vi "Simple Button Lamp Example.vi"() -> ()   [LabVIEW 2018]
uses:
  Lamp/Lamp.lvclass
  Button/Button.lvclass
  Button/Button.lvclass/Button.ctl
  Button/Set Button Pressed.vi
  SwitchableDevice_interface/SwitchableDevice.lvclass
panel:
  out "Lamp":bool
  in  "Button":bool
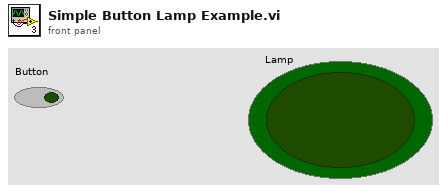
[diagram p1: front panel]
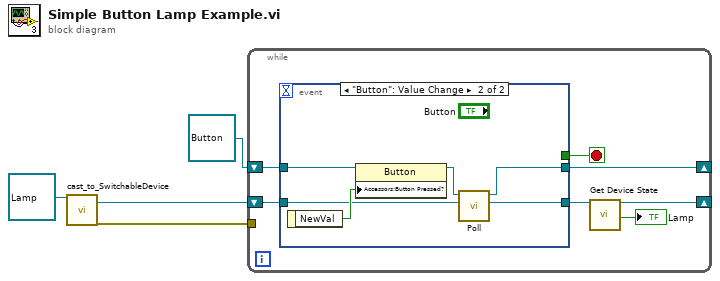
[diagram p0: block diagram]
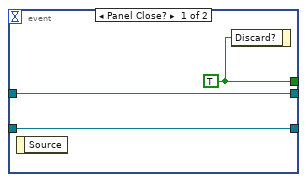
[diagram p2: hidden frame]
diagram:
  n1 = call "cast_to_SwitchableDevice.vi"("Object in"=refnum<class "Lamp.lvclass"> refnum ("Lamp.lvclass")) -> ("Interface_object out"=w2:refnum<class "SwitchableDevice.lvclass">, "error out"=w1:errorcluster)  [unwired: 17 in]
  n2 = while {
    shift-right: [w8] -> _
    shift-left: refnum<class "Button.lvclass"> refnum ("Button in") -> [w10]
    shift-right: [w6] -> _
    shift-left: w2 -> [w9]
    tunnel: w1 -> [_]
    stop <- w11 stop-if-true
    n3 = event shown="[1] \"Button\": Value Change" {
      selector: _ -> [_ _]
      dyn-events: _ -> [_ _]
      timeout: _ -> [_ _]
      tunnel: [w14 _] -> w11
      tunnel: w10 -> [w13 w20]
      tunnel: w9 -> [w12 w17]
      tunnel: [w13 w16] -> w8
      tunnel: [w12 w15] -> w7
      event Panel Close? {
        w14 = TRUE ("Discard?")
        n4 = event-data() -> ()  [unwired: 1 in, 1 out]
        n5 = event-data("Discard?"=w14) -> ()  [unwired: 1 in, 1 out]
      }
      event "Button": Value Change {
        n6 = event-data() -> ("NewVal"=w18:bool)  [unwired: 1 in]
        n7 = property class="Button"(reference=w20, "Accessors:Button Pressed?"=w18) -> (reference out=w19:refnum<class "Button.lvclass">)  [unwired: 1 in, 1 out]
        n8 = call-dynamic "Poll.vi"("Switchable Device in"=w17, "Button in"=w19) -> ("Switchable Device out"=w15:refnum<class "SwitchableDevice.lvclass">, "Button out"=w16:refnum<class "Button.lvclass">)  [unwired: 7 in, 1 out]
      }
    }
    n9 = call "Get Device State.vi"("Interface_object in"=w7) -> ("Interface_object out"=w6:refnum<class "SwitchableDevice.lvclass">, "Device State"=→"Lamp":bool)  [unwired: 16 in, 1 out]
  }
